vi "IFwTest.vi"() -> ()   [LabVIEW 2017]
uses:
  <vilib>/Platform/TimedLoop/XDataNode/timing_clust.ctl
  <vilib>/Platform/TimedLoop/XDataNode/nitl_modes.ctl
  <vilib>/Platform/TimedLoop/XDataNode/wakeup.ctl
  <instrlib>/_niInstr/FIFO Register Bus/v1/FPGA/niInstr FIFO Register Bus v1 FPGA.lvclass
  C:/Program Files (x86)/National Instruments/LabVIEW 2017/instr.lib/_niInstr/Instruction Framework/v1/FPGA/Interfaces/Instruction Producer/Instruction Producer.lvclass
  <instrlib>/_niInstr/Instruction Framework/v1/FPGA/Helper Classes/Single Address Space Collection/Single Address Space Collection.lvclass
  C:/Program Files (x86)/National Instruments/LabVIEW 2017/instr.lib/_niInstr/Instruction Framework/v1/FPGA/Interfaces/Address Space Collection/Address Space Collection.lvclass
  <vilib>/rvi/Emulation/niFpgaGetClockAttributes.vi
  <vilib>/rvi/Emulation/niFpgaSctlEmulationGetInTimedLoop.vi
  <vilib>/rvi/Emulation/niFpgaEmulationReportErrorSimple.vi
  <vilib>/rvi/DataTransferAndStorage/Container/Common/niFpgaContainerExecOnDevCompGetState.vi
  <vilib>/rvi/Emulation/niFpgaEmulationIsFPGAContextNoSignature.vi
  <vilib>/rvi/DataTransferAndStorage/Container/Common/niFpgaContainerGetUniqueNameForEmu.vi
  <vilib>/rvi/Memory/Memory_Emulation/niFpgaMemoryEmulationCacheClearOnFirstRun.vi
  <vilib>/rvi/Memory/Memory_Emulation/nirvimemoryEmulationManagerCache_MakeExclusive.vi
  <vilib>/rvi/Memory/Memory_Emulation/niFpgaMemoryEmulationValidateCache.vi
  <vilib>/rvi/Memory/Memory_Emulation/nirvimemoryEmulationManagerCache_InsertValue.vi
  <vilib>/Utility/error.llb/Clear Errors.vi
  <vilib>/rvi/Memory/Memory_Emulation/nirvimemoryEmulationManagerCache_ReleaseExclusive.vi
  <vilib>/rvi/Memory/Memory_Emulation/nirvimemoryEmulationManagerCache_GetValue.vi
  <vilib>/rvi/Memory/Memory_Emulation/nirvimemoryEmulationManagerCache_SetValue.vi
  <vilib>/rvi/Emulation/niFpgaProcessEmulError.vi
  <vilib>/rvi/Emulation/niFpgaCriticalErrorInLSC.vi
  <vilib>/rvi/DataTransferAndStorage/Container/XNode/niFpgaContainer.xnode
  <vilib>/rvi/DataTransferAndStorage/Register/Emulation/niFpgaRegisterEmulationRefIn.vi
  <vilib>/Platform/TimedLoop/XDataNode/XDataNode.xnode
  AFE/AddressSpace.lvclass
  <instrlib>/_niInstr/Instruction Framework/v1/FPGA/Top Level Bus/Register Configuration/Register Configuration.lvclass
  <vilib>/Platform/TimedLoop/XDataNode/XDNodeRunTimeDep.lvlib
panel:
  out "ManualControls":T1
  out "Parameters":T2
  out "Signals":cluster{"resetPLL":bool, "resetControl":bool}
  out "Setpoints":cluster{"VDCLink":sgl, "DirectedIdSetpt":sgl}
  out "Gains":T3
  out "Range":T4
  in  "fifo reg bus ctrl 0":u32
  out "fifo reg bus status 0":u32
  out "fifo reg bus data 0":u64
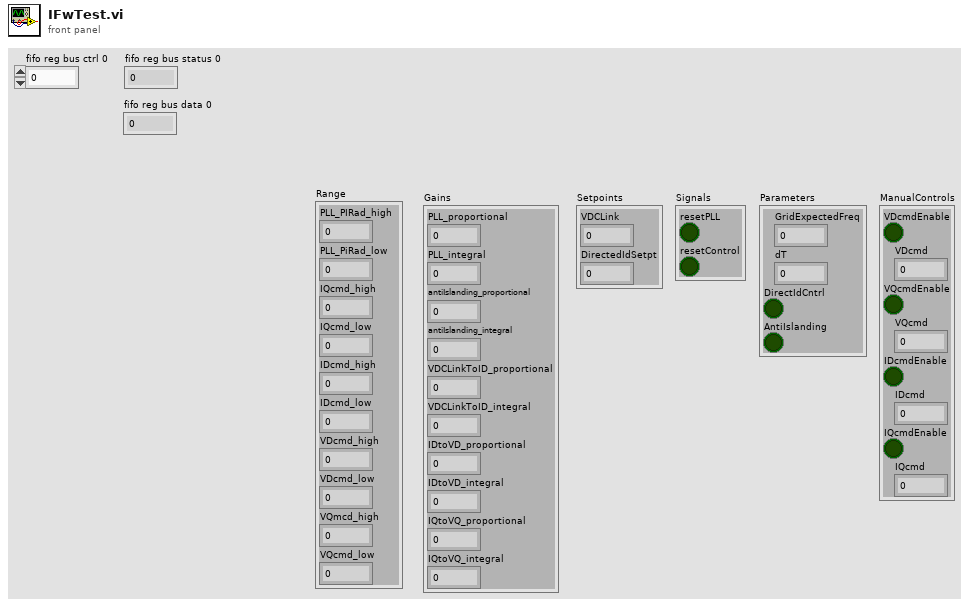
[diagram p1: front panel]
types:
  T1 = cluster{"VDcmdEnable":bool, "VDcmd":sgl, "VQcmdEnable":bool, "VQcmd":sgl, "IDcmdEnable":bool, "IDcmd":sgl, "IQcmdEnable":bool, "IQcmd":sgl}
  T2 = cluster{"GridExpectedFreq":sgl, "dT":sgl, "DirectIdCntrl":bool, "AntiIslanding":bool}
  T3 = cluster{"PLL_proportional":sgl, "PLL_integral":sgl, "antiIslanding_proportional":sgl, "antiIslanding_integral":sgl, "VDCLinkToID_proportional":sgl, "VDCLinkToID_integral":sgl, "IDtoVD_proportional":sgl, "IDtoVD_integral":sgl, "IQtoVQ_proportional":sgl, "IQtoVQ_integral":sgl}
  T4 = cluster{"PLL_PIRad_high":sgl, "PLL_PiRad_low":sgl, "IQcmd_high":sgl, "IQcmd_low":sgl, "IDcmd_high":sgl, "IDcmd_low":sgl, "VDcmd_high":sgl, "VDcmd_low":sgl, "VQmcd_high":sgl, "VQcmd_low":sgl}
  T5 = typedef "XDNodeRunTimeDep.lvlib/timing_clust.ctl" = cluster{"Expected End [f-1]":u64, "Actual End [f-1]":u64, "Finished Late? [f-1]":bool, "Expected End [i-1]":u64, "Actual End [i-1]":u64, "Finished Late? [i-1]":bool, "Expected Start [i]":u64, "Actual Start [i]":u64, "Expected Start [f]":u64, "Actual Start [f]":u64, "Source Name":string, "Structure Name":string, "Period":i64, "Deadline":i64, "Offset":i64, "Start":i64, "Priority":i32, "Timeout":i32, "Mode":T6, "Wakeup Reason":T7, "Error":errorcluster, "Source Type":string, "Secondary Source Type":string, "Global End Time":u64, "Global Start Time":u64, "Frame Duration":u64, "Iteration Duration":u64, "Assigned CPU":i32, "I/O Scan Engine Mode":u32}
  T6 = typedef "XDNodeRunTimeDep.lvlib/nitl_modes.ctl" = enum32{"No Change", "Process missed periods, maintain original phase", "Discard missed periods, maintain original phase", "Process missed periods, ignore original phase", "Discard missed periods, ignore original phase"}
  T7 = typedef "XDNodeRunTimeDep.lvlib/wakeup.ctl" = enum32{"Normal", "Aborted", "Asynchronous wakeup", "Timing source error", "Timed loop error", "Timeout"}
  T8 = typedef "ActiveFrontEnd.lvlib/ControllerRegisters.ctl" = cluster{"Range":refnum<k21>, "Gains":refnum<k21>, "Setpoints":refnum<k21>, "Signals":refnum<k21>, "Parameters":refnum<k21>, "ManualControl":refnum<k21>}
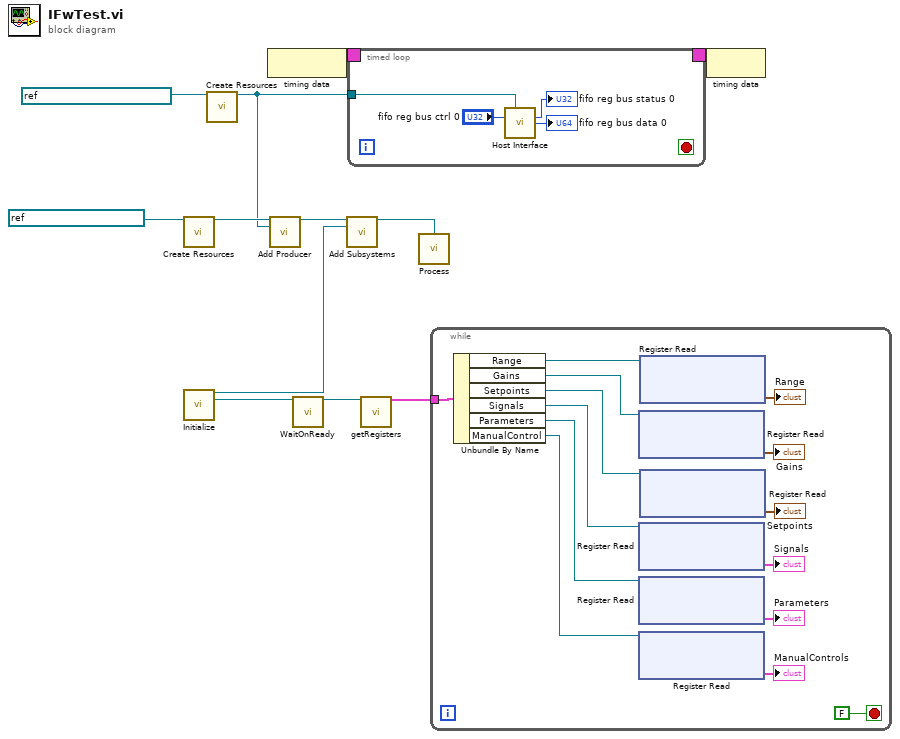
[diagram p0: block diagram]
diagram:
  n1 = call <instrlib>:"Create Resources.vi"("register clock"=refnum<k21> "40 MHz Onboard Clock") -> ("register configuration"=w7:refnum<class "Register Configuration.lvclass">)  [unwired: 14 in]
  n2 = call "Initialize.vi"() -> ("subsysytem"=w4:refnum<class "Single Address Space Collection.lvclass">, "AddressSpace"=w12:refnum<class "AddressSpace.lvclass">)  [unwired: 14 in]
  n3 = call <instrlib>:"Create Resources.vi"("instruction fifo"=refnum<k21> "reg.host instruction fifo 0") -> ("fifo register bus"=w5:refnum<class "niInstr FIFO Register Bus v1 FPGA.lvclass">)  [unwired: 14 in]
  n4 = node-c288() -> (w11:T5)
  n5 = call <instrlib>:"Add Producer.vi"("register configuration in"=w7, "instruction producer"=w5) -> ("register configuration out"=w6:refnum<class "Register Configuration.lvclass">)  [unwired: 13 in]
  n6 = call "WaitOnReady.vi"("AddressSpace in"=w12) -> ("AddressSpace out"=w2:refnum<class "AddressSpace.lvclass">)  [unwired: 14 in]
  n7 = call <instrlib>:"Add Subsystems.vi"("register configuration in"=w6, "subsystems"=w4) -> ("register configuration out"=w3:refnum<class "Register Configuration.lvclass">)  [unwired: 13 in]
  n8 = timed-loop {
    timing: w11 -> [_]
    timing-out: [_] -> w10
    tunnel: w5 -> [w16]
    stop <- _ stop-if-true
    n9 = call <instrlib>:"Host Interface.vi"("fifo register bus"=w16, "fifo reg bus ctrl 0"="fifo reg bus ctrl 0") -> ("fifo reg bus status 0"=→"fifo reg bus status 0":u32, "fifo reg bus data 0"=→"fifo reg bus data 0":u64)  [unwired: 12 in]
  }
  n10 = call "getRegisters.vi"("AddressSpace in"=w2) -> ("CntlRegisters"=w1:T8)  [unwired: 14 in]
  n11 = call <instrlib>:"Process.vi"("register configuration"=w3) -> ()  [unwired: 15 in]
  n12 = while {
    tunnel: w1 -> [w32]
    stop <- FALSE stop-if-true
    n13 = Unbundle By Name(w32) -> ("Range"=w31:refnum<k21>, "Gains"=w30:refnum<k21>, "Setpoints"=w29:refnum<k21>, "Signals"=w28:refnum<k21>, "Parameters"=w27:refnum<k21>, "ManualControl"=w26:refnum<k21>)
    n14 = xnode "Register Read"("Register In"=w30) -> ("Data"=→"Gains":T3)  [unwired: 1 out]
    n15 = xnode "Register Read"("Register In"=w28) -> ("Data"=→"Signals":cluster{"resetPLL":bool, "resetControl":bool})  [unwired: 1 out]
    n16 = xnode "Register Read"("Register In"=w27) -> ("Data"=→"Parameters":T2)  [unwired: 1 out]
    n17 = xnode "Register Read"("Register In"=w26) -> ("Data"=→"ManualControls":T1)  [unwired: 1 out]
    n18 = xnode "Register Read"("Register In"=w31) -> ("Data"=→"Range":T4)  [unwired: 1 out]
    n19 = xnode "Register Read"("Register In"=w29) -> ("Data"=→"Setpoints":cluster{"VDCLink":sgl, "DirectedIdSetpt":sgl})  [unwired: 1 out]
  }
  n20 = node-c288(w10) -> ()
